vi "Write Sync Channel Setting.vi"(8 "error in (no error)":errorcluster, 10 "Sync Channel Setting":T1={"Inverter"=FALSE, "Update Edge"="PXI_Clk100", "Source"="PXI_Clk100", "Type"="PXI_Clk100", "Synchronization Clock"="PXI_Clk100", "Destination"="PXI_Clk100"}, 11 "Sync Channel configuration in":refnum<class "Synchronization Channel configuration.lvclass">) -> (0 "error out":errorcluster, 3 "Sync Channel configuration out":refnum<class "Synchronization Channel configuration.lvclass">)   [LabVIEW 2025, in "Synchronization.lvlib" / "Synchronization Channel configuration.lvclass"]
uses:
  Synchronization Channel configuration.lvclass
  Synchronization Channel configuration.lvclass/Synchronization Channel configuration.ctl
  Sync Channel Setting.ctl
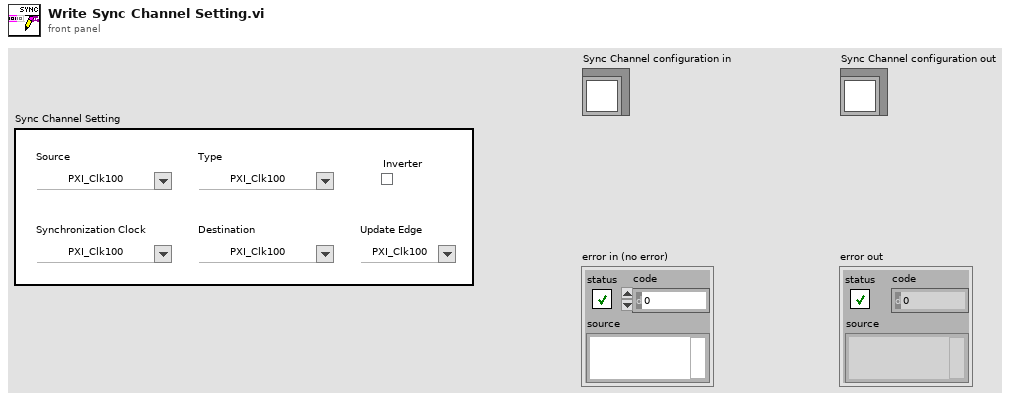
[diagram p1: front panel]
types:
  T1 = typedef "Synchronization.lvlib/Synchronization Channel configuration.lvclass/Sync Channel Setting.ctl" = cluster{"Inverter":bool, "Update Edge":string, "Source":string, "Type":string, "Synchronization Clock":string, "Destination":string}
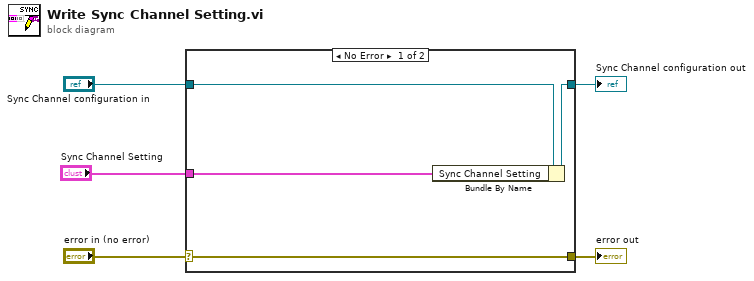
[diagram p0: block diagram]
diagram:
  n1 = case shown="No Error" "error in (no error)" {
    selector: "error in (no error)" -> [w9 w10]
    tunnel: [w9 w10] -> w4
    tunnel: [w7 w11] -> w2
    tunnel: "Sync Channel configuration in" -> [w8 w11]
    tunnel: "Sync Channel Setting" -> [w6 _]
    frame No Error {
      n2 = Bundle By Name(cluster=w8, "Sync Channel Setting"=w6) -> (w7:refnum<class "Synchronization Channel configuration.lvclass">)
    }
    frame Error {
    }
  }
  "error out" <- w4
  "Sync Channel configuration out" <- w2
